vi "ExecutePauseMusicCommand.vi"(0 "reference in":refnum<class "RemoteControl.lvclass">, 11 "Error In":errorcluster) -> (4 "reference out":refnum<class "RemoteControl.lvclass">, 15 "Error Out":errorcluster)   [LabVIEW 2024, in "RemoteControl.lvclass"]
uses:
  RemoteControl.lvclass
  RemoteControl.lvclass/RemoteControl.ctl
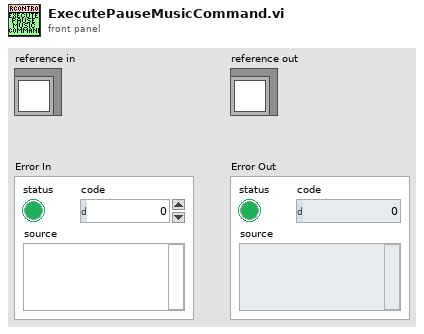
[diagram p1: front panel]
types:
  T1 = typedef "RemoteControl.lvclass/ObjectAttributes.ctl" = cluster{"PlayMusicCommand":refnum<class "IPlayerCommand.lvclass">, "PauseMusicCommand":refnum<class "IPlayerCommand.lvclass">, "StopMusicCommand":refnum<class "IPlayerCommand.lvclass">, "SkipMusicCommand":refnum<class "IPlayerCommand.lvclass">}
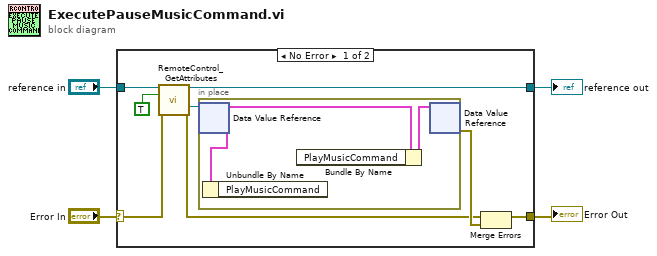
[diagram p0: block diagram]
diagram:
  n1 = case shown="No Error" "Error In" {
    selector: "Error In" -> [w11 w16]
    tunnel: [w8 w16] -> w3
    tunnel: [w9 w15] -> w1
    tunnel: "reference in" -> [w12 w15]
    frame No Error {
      n2 = call "RemoteControl_GetAttributes.vi"("reference in"=w12, "OnlyGetDvrReference(False)"=TRUE, "Error In"=w11) -> ("reference out"=w9:refnum<class "RemoteControl.lvclass">, "DataRef"=w7:refnum<data-value>, "Error Out"=w6:errorcluster)  [unwired: 9 in, 1 out]
      n3 = in-place {
        n4 = in-place-dvr #1(w7) -> (w13:T1)  [unwired: 1 out]
        n5 = Unbundle By Name(w13) -> ()  [unwired: 1 out]
        n6 = Bundle By Name(cluster=w13) -> (w14:T1)  [unwired: 1 in]
        n7 = in-place-dvr #1(w14) -> (w10:errorcluster)  [unwired: 1 out]
      }
      n8 = Merge Errors(w6, w10) -> (w8:errorcluster)
    }
    frame Error {
    }
  }
  "Error Out" <- w3
  "reference out" <- w1
